vi "string to key-value.vi"(4 "separation between key and value":string=":", 5 "separation between K-V sections":string=";", 6 "known key list":string[](array[string])=["SET_PID", "SET_OUTPUT"], 7 "input string":string) -> (1 "key index list":i32[](array[numeric]), 2 "value list":string[](array[string]), 3 "key list":string[](array[string]))   [LabVIEW 2018]
uses:
  <vilib>/Utility/error.llb/whitespace.ctl
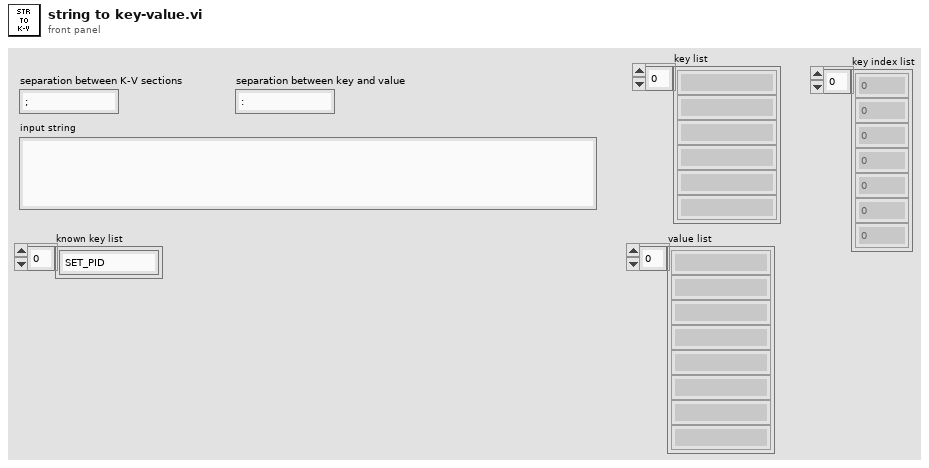
[diagram p1: front panel]
types:
  T1 = typedef "whitespace.ctl" = u16
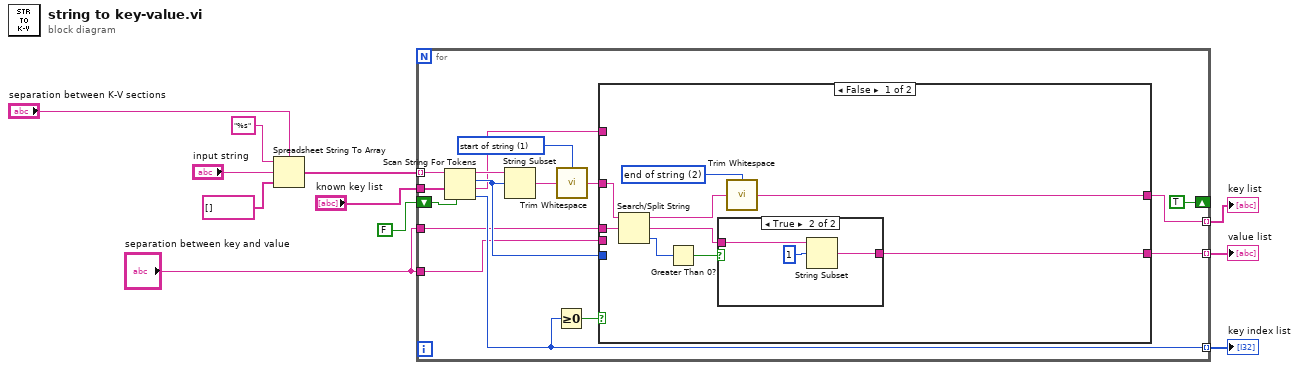
[diagram p0: block diagram]
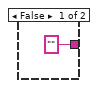
[diagram p2: hidden frame]
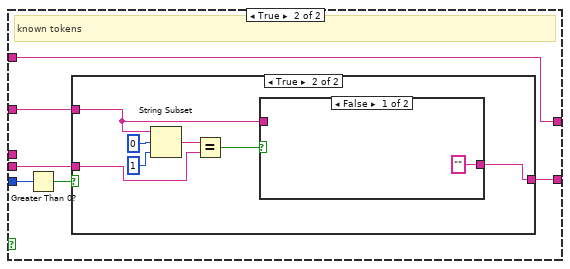
[diagram p3: hidden frame]
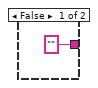
[diagram p4: hidden frame]
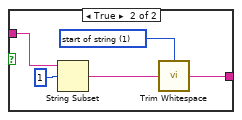
[diagram p5: hidden frame]
diagram:
  n1 = Spreadsheet String To Array(delimiter (Tab)="separation between K-V sections", format string="%s", spreadsheet string="input string", array type (2D Dbl)=string[] []) -> (array=w7:string[])
  n2 = for {
    shift-right: [TRUE] -> _
    shift-left: FALSE -> [w27]
    tunnel: w7 -> [w25] mode=indexing
    tunnel: "known key list" -> [w24]
    tunnel: [w22] -> w4 mode=indexing
    tunnel: [w12] -> w5 mode=indexing
    tunnel: [w17] -> w6 mode=indexing
    tunnel: "separation between key and value" -> [w15]
    tunnel: "separation between key and value" -> [w14]
    w20 = T1 1 items=["both", "start of string", "end of string"] ("location (both)")
    n3 = Scan String For Tokens(4:w27, 7:w24, 9:w25) -> (0:w22:i32, 1:w13:string, 2:w16:i32, 3:w19:string)  [unwired: 3 in]
    n4 = String Subset(string=w19, offset (0)=w16) -> (substring=w21:string)  [unwired: 1 in]
    n5 = Greater Or Equal To 0?(x=w22) -> (x >= 0?=w23:bool)
    n6 = call <vilib>:"Trim Whitespace.vi"("string"=w21, "location (both)"=w20) -> ("trimmed string"=w18:string)
    n7 = case shown="False" w23 {
      tunnel: w18 -> [w36 w45]
      tunnel: [w28 w44] -> w17
      tunnel: w16 -> [_ w43]
      tunnel: w15 -> [_ w46]
      tunnel: w14 -> [w34 _]
      tunnel: [w33 w41] -> w12
      tunnel: w13 -> [_ w41]
      frame False {
        w32 = T1 2 items=["both", "start of string", "end of string"] ("location (both)")
        n8 = Search/Split String(string=w36, search string/char (-)=w34) -> (substring before match=w35:string, match + rest of string=w31:string, offset of match=w30:i32)  [unwired: 1 in]
        n9 = Greater Than 0?(x=w30) -> (x > 0?=w29:bool)
        n10 = case shown="True" w29 {
          tunnel: w31 -> [_ w40]
          tunnel: ["" ("trimmed string") w38] -> w28
          frame False {
          }
          frame True {
            n11 = String Subset(string=w40, offset (0)=1) -> (substring=w38:string)  [unwired: 1 in]
          }
        }
        n12 = call <vilib>:"Trim Whitespace.vi"("string"=w35, "location (both)"=w32) -> ("trimmed string"=w33:string)
      }
      frame True {
        # "known tokens"
        n13 = Greater Than 0?(x=w43) -> (x > 0?=w42:bool)
        n14 = case shown="True" w42 {
          tunnel: w46 -> [_ w51]
          tunnel: w45 -> [_ w49]
          tunnel: ["" ("trimmed string") w48] -> w44
          frame False {
          }
          frame True {
            n15 = String Subset(string=w49, offset (0)=0, length (rest)=1 ("length (rest)")) -> (substring=w52:string)
            n16 = Equal?(x=w52, y=w51) -> (x = y?=w50:bool)
            n17 = case shown="False" w50 {
              tunnel: w49 -> [_ w60]
              tunnel: ["" ("trimmed string") w57] -> w48
              frame False {
              }
              frame True {
                w56 = T1 1 items=["both", "start of string", "end of string"] ("location (both)")
                n18 = String Subset(string=w60, offset (0)=1) -> (substring=w58:string)  [unwired: 1 in]
                n19 = call <vilib>:"Trim Whitespace.vi"("string"=w58, "location (both)"=w56) -> ("trimmed string"=w57:string)
              }
            }
          }
        }
      }
    }
  }
  "value list" <- w6
  "key list" <- w5
  "key index list" <- w4
